vi "serial_05.vi"(0 "VISA":refnum<visa-resource-name>="COM5") -> ()   [LabVIEW 2009]
doc: "The Basic Serial Read and Write example performs a Serial Port Read, a Serial Port Write, or a combination of these actions. The user selects the actions (read or write) on the front panel. If both are selected, the VI will write the data first, read data, and then close the VISA session that is opened to the port. This VI will wait until the specified number of bytes is received at the port. Only the number of bytes specified will be read.\n\nINSTRUCTIONS:\n1) Select the serial resource and configuration parameters (baud rate, data bits, parity, stop bits, flow control).\n2) Select the operations to be performed. \n3) Connect the serial port to your device. If no device is available, perform a loopback test by doing one of the following. Short pins 2 and 3 on a RS-232 cable or short pin 4 to pin 8 and pin 5 to pin 9 on a RS-485/422 cable. \n4) Run the VI to see the data read. (The \"read string\" will match the \"string to write\" if a loopback test was performed.)\n\nNote: The parameters set for the serial port must match the parameters of the connected instrument or device. In this example, the bytes to read parameter specifies the number of bytes that the serial port reads. If there were more bytes at the port than the number specified in bytes to read, those bytes would not be read. Also, if you specify to read more bytes than the number of bytes actually read, you might receive a timeout error message.\n\nOn the block diagram, the Configure Serial Port VI sets the configuration parameters. The front panel displays the controls used to configure the basic parameters, such as baud rate, data bits, and parity. Constants configure the other parameters the user probably does not need set. After the VISA Configure Serial Port VI opens the VISA session and configures the port, the VI passes the VISA resource name to other VIs that perform operations on that VISA resource. The VISA Write function sends a command to the serial device and the VISA Read function returns data based on the command. The VISA Close function then closes the reference to the serial device. It is important to close the reference; otherwise communication through with that port through protocols other than VISA might not be possible."
panel:
  out "A4":string
  out "A3":string
  out "A2":string
  out "A1":string
  out "A0":string
  out "String":string
  in  "Start":bool=TRUE
  # "Stop"
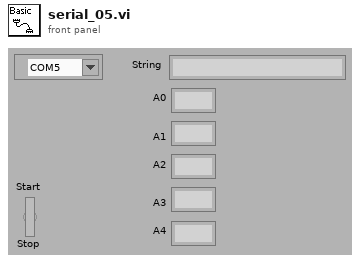
[diagram p1: front panel]
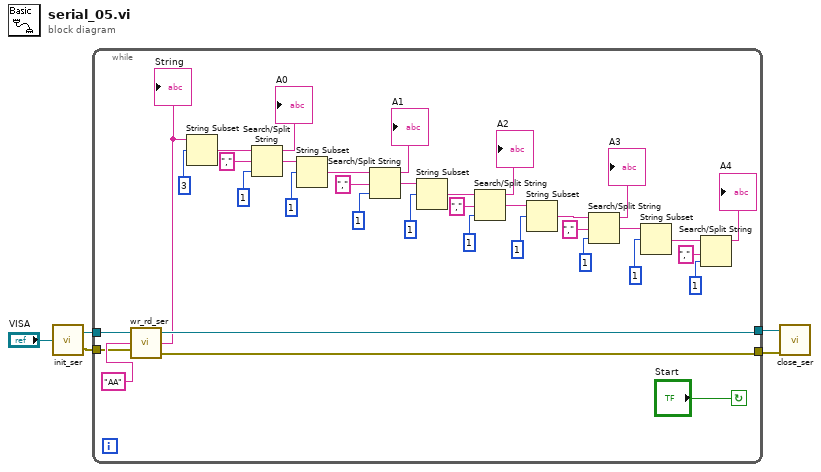
[diagram p0: block diagram]
diagram:
  n1 = call "init_ser.vi"("VISA resource name"="VISA") -> ("VISA resource name out"=w3:refnum<visa-resource-name>, "error out"=w4:errorcluster)
  n2 = while {
    tunnel: w4 -> [w38]
    tunnel: w3 -> [w39]
    tunnel: [w36] -> w2
    tunnel: [w37] -> w1
    stop <- "Start" continue-if-true
    n3 = call "wr_rd_ser.vi"("error in"=w38, "string to write"="AA", "VISA resource name in"=w39) -> ("error out"=w36:errorcluster, "read buffer"=w25:string, "VISA resource name out"=w37:refnum<visa-resource-name>)
    "String" <- w25
    n4 = String Subset(string=w25, offset (0)=3) -> (substring=w24:string)  [unwired: 1 in]
    n5 = Search/Split String(string=w24, search string/char (-)=",", offset (0)=1) -> (substring before match=→"A0":string, match + rest of string=w29:string)  [unwired: 1 out]
    n6 = String Subset(string=w29, offset (0)=1) -> (substring=w27:string)  [unwired: 1 in]
    n7 = Search/Split String(string=w27, search string/char (-)=",", offset (0)=1 ("x")) -> (substring before match=→"A1":string, match + rest of string=w18:string)  [unwired: 1 out]
    n8 = String Subset(string=w18, offset (0)=1) -> (substring=w19:string)  [unwired: 1 in]
    n9 = Search/Split String(string=w19, search string/char (-)=",", offset (0)=1 ("x")) -> (substring before match=→"A2":string, match + rest of string=w12:string)  [unwired: 1 out]
    n10 = String Subset(string=w12, offset (0)=1) -> (substring=w14:string)  [unwired: 1 in]
    n11 = Search/Split String(string=w14, search string/char (-)=",", offset (0)=1 ("x")) -> (substring before match=→"A3":string, match + rest of string=w7:string)  [unwired: 1 out]
    n12 = String Subset(string=w7, offset (0)=1) -> (substring=w8:string)  [unwired: 1 in]
    n13 = Search/Split String(string=w8, search string/char (-)=",", offset (0)=1 ("x")) -> (substring before match=→"A4":string)  [unwired: 2 out]
  }
  n14 = call "close_ser.vi"("error in"=w2, "VISA resource name in"=w1) -> ()
